vi "process_DAQ_NI.vi"(8 "error in (no error)":errorcluster) -> (0 "error out":errorcluster)   [LabVIEW 2010]
uses:
  typedefs/control_daq_enum.ctl
  typedefs/data_array.ctl
  typedefs/acquisition_parameters_NI_cluster.ctl
  typedefs/device_parameters.ctl
  typedefs/protocol_parameters.ctl
  <vilib>/DAQmx/read.llb/DAQmx Read (Analog 1D Wfm NChan NSamp).vi
  <vilib>/daqmx/miscellaneous.llb/DAQmx Fill In Error Info.vi
panel:
  out "Acquiring":bool
  out "Package start time":timestamp format="%<%.3X>T"
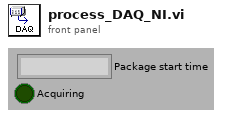
[diagram p1: front panel]
types:
  T1 = typedef "control_daq_enum.ctl" = enum16{"Init", "GetCont", "GetNoSamples", "Stop", "Quit"}
  T2 = cluster{"Control DAQ Enum":T1, "variant":variant}
  T3 = typedef "data_array.ctl" = waveform(dbl)[]
  T4 = typedef "acquisition_parameters_NI_cluster.ctl" = cluster{"Physical channels":tag, "Shutter line":tag, "Triggered?":bool, "Sample rate":dbl, "Pixels to integrate":i32, "Effective data rate":dbl, "Read chunk size":i32, "Samples to read":i32, "Run mode":enum32{"Continuously", "Fixed sample number"}}
  T5 = typedef "device_parameters.ctl" = cluster{"Triggered?":bool, "Shutter channel":tag, "Acquisition channels":tag, "Acquisition sample rate":dbl, "Pixels to integrate":i32, "Effective sample rate":dbl, "Read chunk size":i32, "Stimulation channel":tag, "Stimulation sample rate":dbl}
  T6 = typedef "protocol_parameters.ctl" = cluster{"Repetitions":dbl, "ON time":dbl, "OFF time":dbl, "Stim onset":dbl, "Stim frequency":dbl, "Stim length":dbl, "Acquire before ON":dbl, "Acquire after ON":dbl, "Sync shutter to acquisition":bool}
  T7 = cluster{"Device parameters":T5, "Protocol parameters":T6}
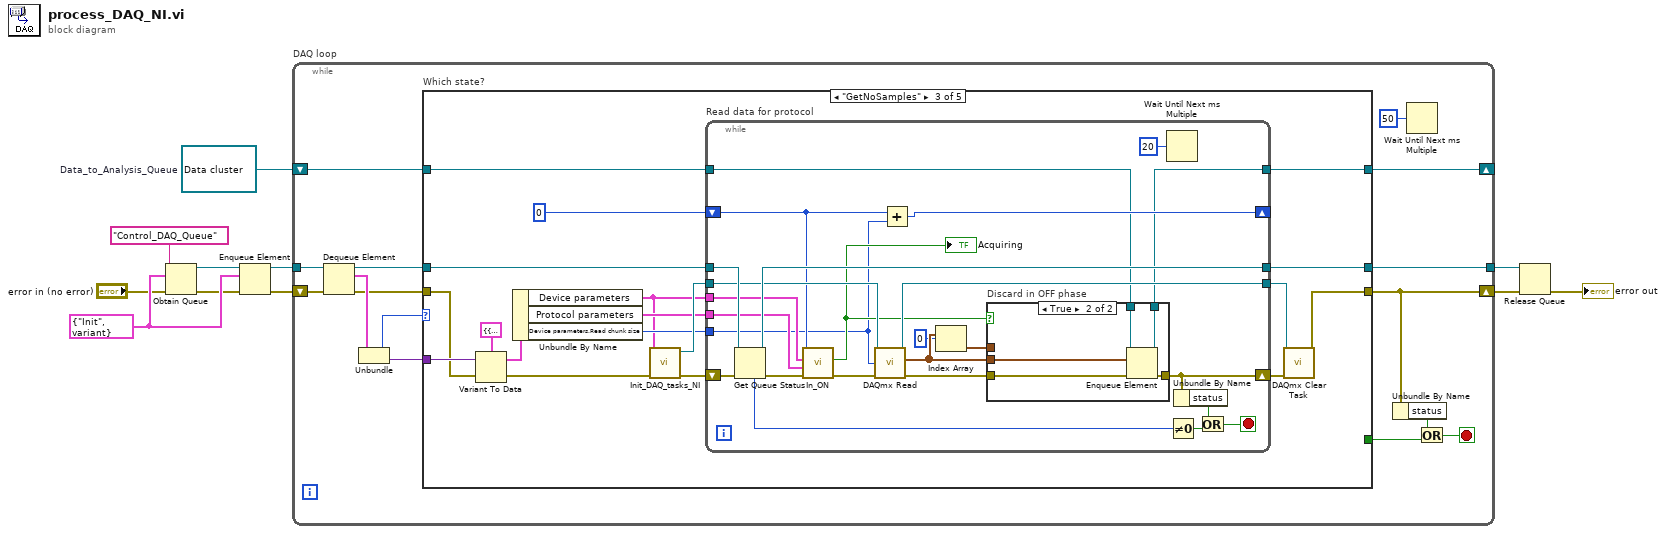
[diagram p0: block diagram]
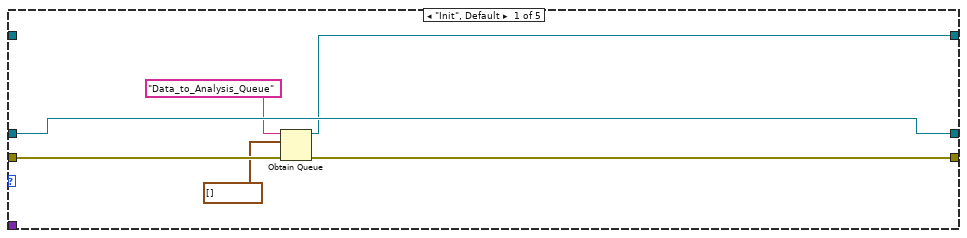
[diagram p2: hidden frame]
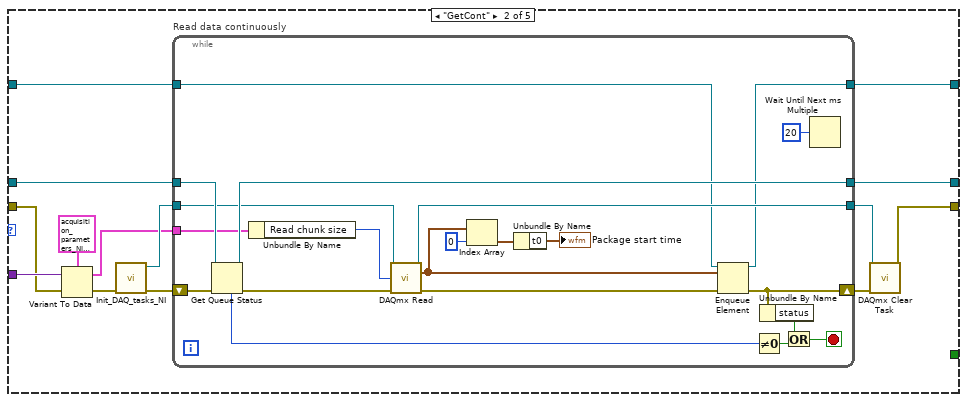
[diagram p3: hidden frame]
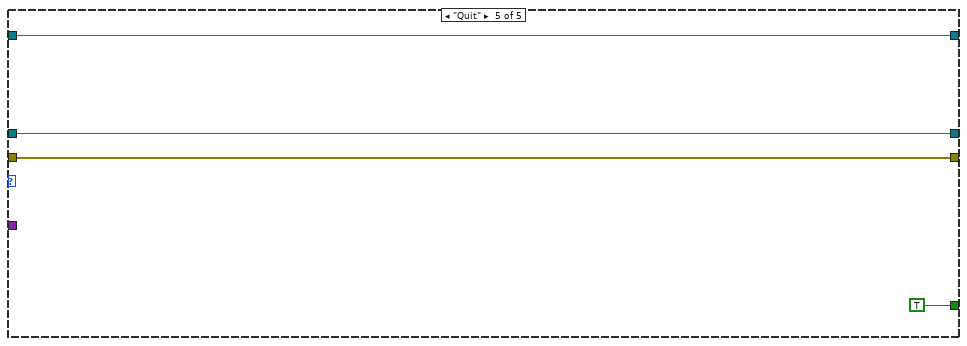
[diagram p6: hidden frame]
diagram:
  w1 = refnum<queue> refnum  # Data_to_Analysis_Queue
  w11 = T2 {"Control DAQ Enum"=enum."Init", "variant"=variant} ("ControlDAQ state cluster")
  n1 = Obtain Queue(name (unnamed)="Control_DAQ_Queue", element data type=w11, error in (no error)="error in (no error)") -> (queue out=w7:refnum<queue>, error out=w9:errorcluster)  [unwired: 2 in, 1 out]
  n2 = Enqueue Element(queue=w7, element=w11, error in (no error)=w9) -> (queue out=w8:refnum<queue>, error out=w10:errorcluster)  [unwired: 1 in, 1 out]
  n3 = while "DAQ loop" {
    shift-right: [w19] -> w6
    shift-left: w10 -> [w25]
    tunnel: w8 -> [w26]
    tunnel: [w15] -> w5
    shift-right: [w12] -> _
    shift-left: w1 -> [w13]
    stop <- w17 stop-if-true
    n4 = Dequeue Element(queue=w26, error in (no error)=w25) -> (queue out=w24:refnum<queue>, element=w23:T2, error out=w21:errorcluster)  [unwired: 1 in, 1 out]
    n5 = Unbundle(w23) -> ("Control DAQ Enum"=w16:T1, "variant"=w22:variant)
    n6 = case "Which state?" shown="\"GetNoSamples\"" w16 {
      tunnel: w24 -> [w32 w46 w85 w119 w122]
      tunnel: w22 -> [_ w45 w84 _ _]
      tunnel: w21 -> [w31 w44 w83 w120 w123]
      tunnel: [w29 w37 w76 w120 w123] -> w19
      tunnel: [_ _ _ _ TRUE] -> w20
      tunnel: [w32 w43 w82 w119 w122] -> w15
      tunnel: w13 -> [_ w34 w73 w118 w121]
      tunnel: [w27 w33 w72 w118 w121] -> w12
      frame "Init", Default {
        n7 = Obtain Queue(name (unnamed)="Data_to_Analysis_Queue", element data type=T3 [] ("Data cluster"), error in (no error)=w31) -> (queue out=w27:refnum<queue>, error out=w29:errorcluster)  [unwired: 2 in, 1 out]
      }
      frame "GetCont" {
        n8 = Variant To Data(error in=w44, Variant=w45, type=T4 {"Physical channels"="", "Shutter line"="", "Triggered?"=FALSE, "Sample rate"=1000.0, "Pixels to integrate"=10, "Effective data rate"=0.0, "Read chunk size"=100, "Samples to read"=2000, "Run mode"=enum."Continuously"} ("Acquisition parameters")) -> (error out=w40:errorcluster, data=w36:T4)
        n9 = call "Init_DAQ_tasks_NI.vi"("error in"=w40) -> ("error out"=w42:errorcluster, "DAQ task out"=w41:refnum<k21>)  [unwired: 7 in]
        n10 = while "Read data continuously" {
          shift-right: [w61] -> w39
          shift-left: w42 -> [w62]
          tunnel: w46 -> [w67]
          tunnel: [w63] -> w43
          tunnel: w41 -> [w57]
          tunnel: w36 -> [w51]
          tunnel: [w49] -> w38
          tunnel: w34 -> [w48]
          tunnel: [w47] -> w33
          stop <- w64 stop-if-true
          n11 = Get Queue Status(queue=w67, error in (no error)=w62) -> (queue out=w63:refnum<queue>, error out=w50:errorcluster, # elements in queue=w66:i32)  [unwired: 1 in, 5 out]
          n12 = Unbundle By Name(w51) -> ("Read chunk size"=w58:i32)
          n13 = call-poly <vilib>:"DAQmx Read.vi"("task/channels in"=w57, "number of samples per channel"=w58, "error in"=w50) -> ("task out"=w49:refnum<k21>, "data"=w55:waveform(dbl)[], "error out"=w56:errorcluster)  [unwired: 10 in]
          n14 = Index Array(array=w55, index=0) -> (element=w53:waveform(dbl))
          n15 = Unbundle By Name(w53) -> ("t0"=→"Package start time":timestamp)
          n16 = Enqueue Element(queue=w48, element=w55, error in (no error)=w56) -> (queue out=w47:refnum<queue>, error out=w61:errorcluster)  [unwired: 1 in, 1 out]
          n17 = Not Equal To 0?(x=w66) -> (x != 0?=w65:bool)
          n18 = Unbundle By Name(w61) -> ("status"=w60:bool)
          n19 = Or(x=w60, y=w65) -> (x .or. y?=w64:bool)
          n20 = Wait Until Next ms Multiple(millisecond multiple=u32 20) -> ()  [unwired: 1 out]
        }
        n21 = call <vilib>:"DAQmx Clear Task.vi"("task in"=w38, "error in"=w39) -> ("error out"=w37:errorcluster)  [unwired: 13 in]
      }
      frame "GetNoSamples" {
        n22 = Variant To Data(error in=w83, Variant=w84, type=T7 {"Device parameters"={"Triggered?"=FALSE, "Shutter channel"="", "Acquisition channels"="", "Acquisition sample rate"=100.0, "Pixels to integrate"=0, "Effective sample rate"=100.0, "Read chunk size"=0, "Stimulation channel"="", "Stimulation sample rate"=100.0}, "Protocol parameters"={"Repetitions"=1.0, "ON time"=40.0, "OFF time"=120.0, "Stim onset"=5.0, "Stim frequency"=1.0, "Stim length"=1.0, "Acquire before ON"=1.0, "Acquire after ON"=0.0, "Sync shutter to acquisition"=FALSE}}) -> (error out=w79:errorcluster, data=w71:T7)
        n23 = Unbundle By Name(w71) -> ("Device parameters"=w68:T5, "Protocol parameters"=w70:T6, "Device parameters.Read chunk size"=w69:i32)
        n24 = call "Init_DAQ_tasks_NI.vi"("error in"=w79, "Device parameters"=w68) -> ("error out"=w81:errorcluster, "DAQ task out"=w80:refnum<k21>)  [unwired: 6 in]
        n25 = while "Read data for protocol" {
          shift-right: [w93] -> w78
          shift-left: w81 -> [w105]
          tunnel: w85 -> [w110]
          tunnel: [w106] -> w82
          tunnel: w80 -> [w103]
          tunnel: [w102] -> w77
          shift-right: [w101] -> _
          shift-left: 0 -> [w100]
          tunnel: w73 -> [w99]
          tunnel: [w98] -> w72
          tunnel: w68 -> [w91]
          tunnel: w70 -> [w90]
          tunnel: w69 -> [w89]
          stop <- w107 stop-if-true
          n26 = Get Queue Status(queue=w110, error in (no error)=w105) -> (queue out=w106:refnum<queue>, error out=w97:errorcluster, # elements in queue=w109:i32)  [unwired: 1 in, 5 out]
          n27 = call "In_ON.vi"("error in"=w97, "Protocol parameters"=w90, "Device parameters"=w91, "Read position"=w100) -> ("error out"=w96:errorcluster, "Do acquire"=w92:bool)  [unwired: 6 in]
          "Acquiring" <- w92
          n28 = call-poly <vilib>:"DAQmx Read.vi"("task/channels in"=w103, "number of samples per channel"=w89, "error in"=w96) -> ("task out"=w102:refnum<k21>, "data"=w88:waveform(dbl)[], "error out"=w95:errorcluster)  [unwired: 10 in]
          n29 = Add(x=w100, y=w89) -> (x+y=w101:i32)
          n30 = Index Array(array=w88, index=0) -> (element=w86:waveform(dbl))
          n31 = case "Discard in OFF phase" shown="True" w92 {
            tunnel: w95 -> [w112 w115]
            tunnel: w99 -> [w111 w117]
            tunnel: [w111 w116] -> w98
            tunnel: [w112 w114] -> w93
            tunnel: w88 -> [_ w113]
            tunnel: w86 -> [_ _]
            frame False {
            }
            frame True {
              n32 = Enqueue Element(queue=w117, element=w113, error in (no error)=w115) -> (queue out=w116:refnum<queue>, error out=w114:errorcluster)  [unwired: 1 in, 1 out]
            }
          }
          n33 = Wait Until Next ms Multiple(millisecond multiple=u32 20) -> ()  [unwired: 1 out]
          n34 = Not Equal To 0?(x=w109) -> (x != 0?=w108:bool)
          n35 = Unbundle By Name(w93) -> ("status"=w94:bool)
          n36 = Or(x=w94, y=w108) -> (x .or. y?=w107:bool)
        }
        n37 = call <vilib>:"DAQmx Clear Task.vi"("task in"=w77, "error in"=w78) -> ("error out"=w76:errorcluster)  [unwired: 13 in]
      }
      frame "Stop" {
      }
      frame "Quit" {
      }
    }
    n38 = Unbundle By Name(w19) -> ("status"=w18:bool)
    n39 = Wait Until Next ms Multiple(millisecond multiple=u32 50) -> ()  [unwired: 1 out]
    n40 = Or(x=w18, y=w20) -> (x .or. y?=w17:bool)
  }
  n41 = Release Queue(queue=w5, error in (no error)=w6) -> (error out=→"error out":errorcluster)  [unwired: 1 in, 2 out]
